vi "CAN ISA Read.vi"() -> (1 "Error Number":u32 format="%.0x", 2 "RcvQueueEmpty":bool, 3 "CAN_Message out":T1 {"ID" format="%.0x"})   [LabVIEW 2009]
doc: "Liest eine Nachricht aus der Queue des Treibers aus. Die Variable RcvQueueEmpty signalisiert das die Queue leer ist."
uses:
  PCAN_ISA.dll
panel:
  in  "CAN_Message":T1={"ID"=0, "MSG type"=enum."STD, NO RTR", "LEN"=0, "DATA"=[0, 0, 0, 0, 0, 0, 0, 0]} {"ID" format="%.0x"}
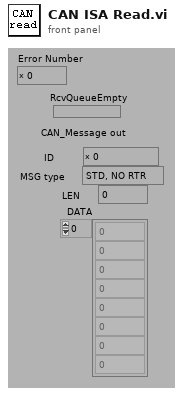
[diagram p1: front panel]
types:
  T1 = cluster{"ID":u32, "MSG type":enum8{"STD, NO RTR", "STD,RTR", "XTD, NO RTR", "XTD, RTR"}, "LEN":u8, "DATA":u8[]}
  T2 = cluster{"ID":u32, "MSG type":enum16{"STD, NO RTR", "STD,RTR", "XTD, NO RTR", "XTD, RTR"}, "LEN":u8, "DATA":u8[]}
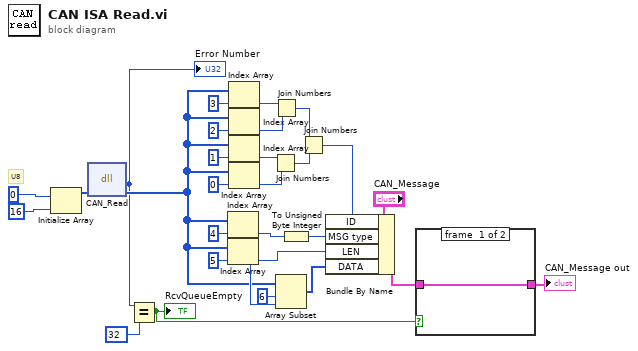
[diagram p0: block diagram]
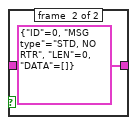
[diagram p2: hidden frame]
diagram:
  # "U8"
  n1 = Initialize Array(u8 0 ("Element Data"), 16 ("Dimension Size")) -> (w6:u8[])
  n2 = dll-call lib="C:/Documents and Settings/PQ/Desktop/LabView-Dateien/PCAN_ISA.dll" fn="CAN_Read"("pMsgBuff"=w6) -> ("Error Number"=w3:u32, "pMsgBuff"=w5:u8[])  [unwired: 3 in, 2 out]
  "Error Number" <- w3
  n3 = Equal?(x=w3, y=i16 32 ("err")) -> (x = y?=w2:bool)
  "RcvQueueEmpty" <- w2
  n4 = Index Array(array=w5, index=4 ("Index")) -> (element=w10:u8)
  n5 = Index Array(array=w5, index=5 ("Index")) -> (element=w11:u8)
  n6 = Index Array(array=w5, index=3 ("Index")) -> (element=w21:u8)
  n7 = Index Array(array=w5, index=2 ("Index")) -> (element=w22:u8)
  n8 = Index Array(array=w5, index=1 ("Index")) -> (element=w20:u8)
  n9 = Index Array(array=w5, index=0 ("Index")) -> (element=w19:u8)
  n10 = Join Numbers(hi=w20, lo=w19) -> ((hi.lo)=w23:u16)
  n11 = Join Numbers(hi=w21, lo=w22) -> ((hi.lo)=w24:u16)
  n12 = Array Subset(array=w5, index=6 ("Array Index"), length=w11) -> (w12:u8[])
  n13 = To Unsigned Byte Integer(number=w10) -> (unsigned 8bit integer=w26:u8)
  n14 = Join Numbers(hi=w24, lo=w23) -> ((hi.lo)=w25:u32)
  n15 = Bundle By Name(cluster="CAN_Message", "ID"=w25, "MSG type"=w26, "LEN"=w11, "DATA"=w12) -> (w18:T1)
  n16 = case shown="True" w2 {
    tunnel: w18 -> [w29 _]
    tunnel: [w29 T2 {"ID"=0, "MSG type"=enum."STD, NO RTR", "LEN"=0, "DATA"=[]} ("CAN_Message out")] -> w1
    frame #0 {
    }
    frame #1 {
    }
  }
  "CAN_Message out" <- w1
